vi "Test In-Range ARGB Image.vi"(8 "error in (no error)":errorcluster, 11 "Test Case In":refnum<class "01_Image.lvclass">) -> (0 "error out":errorcluster, 3 "Test Case Out":refnum<class "01_Image.lvclass">)   [LabVIEW 2020, in "test.lvlib" / "01_Image.lvclass"]
uses:
  01_Image.lvclass
  C:/Program Files (x86)/National Instruments/LabVIEW 2026/vi.lib/Astemes/LUnit/Test Case.lvclass
  common/Image Size (Integer).ctl
  image/In-Range Image Colour Range.ctl
  <vilib>/Astemes/LUnit/Test Case.lvclass/Test Case.ctl
  image/New Image (Greyscale Preallocated).vi
  4993e8ee-a06a-463a-9684-69129f64d5ce.vi
  image/New Image (ARGB Preallocated).vi
  image/Copy Array to Image.vi
  image/Copy Array to Image (ARGB).vi
  image/New Image (Greyscale Preallocated).vi/6598b9e0-8a08-46f5-91fd-ca1b87217137.vi
  image/In-Range (ARGB).vi/ffccc43a-a069-4092-9152-56f2c6e40fec.vi
  <vilib>/Astemes/LUnit/Core/LUnit Test Case/Private/Append Pass Result.vi
  <vilib>/Astemes/LUnit/Core/LUnit Test Case/Private/Append Fail Result.vi
  4993e8ee-a06a-463a-9684-69129f64d5ce.vi/9c5d11cd-9439-4240-a1ee-d9baace9c924.vi
  image/New Image (ARGB Preallocated).vi/3321fa97-f432-4e1e-8db9-a0df79aed21b.vi
  image/ARGB Colour to U32 Pixel Value.vi
  <vilib>/Astemes/LUnit/Core/LUnit Test Case/Private/Run In UI.vi
  <vilib>/Utility/error.llb/Clear Errors.vi
  <vilib>/Utility/error.llb/Error Cluster From Error Code.vi
  <vilib>/picture/pixmap.llb/Flatten Pixmap.vi
  image/image.lvlib
  common/common.lvlib
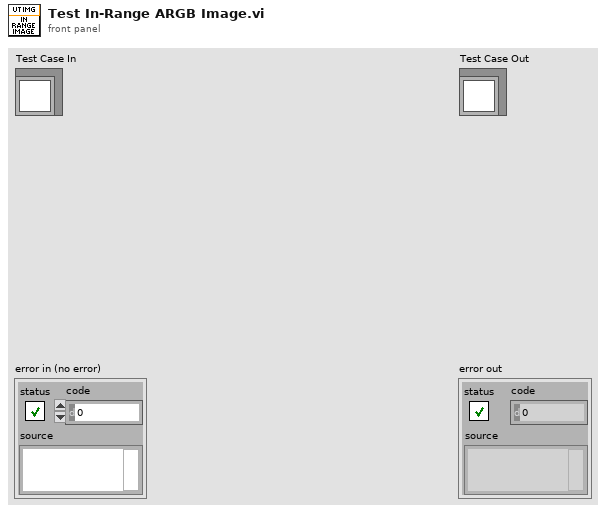
[diagram p1: front panel]
types:
  T1 = typedef "image.lvlib/In-Range Image Colour Range.ctl" = cluster{"Lower":u32, "Upper":u32}
  T2 = typedef "common.lvlib/Image Size (Integer).ctl" = cluster{"Width":u16, "Height":u16}
  T3 = typedef "image.lvlib/ARGB Image.ctl" = refnum<data-value>
  T4 = typedef "image.lvlib/Greyscale Image.ctl" = refnum<data-value>
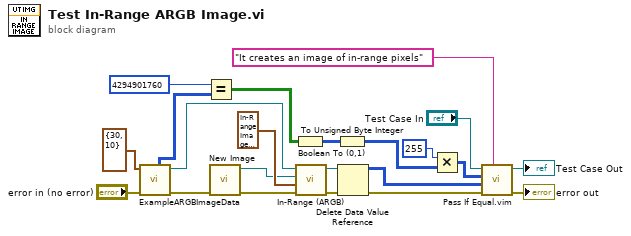
[diagram p0: block diagram]
diagram:
  n1 = call "ExampleARGBImageData.vi"("error in (no error)"="error in (no error)", "Image Size"=T2 {"Width"=30, "Height"=10} ("Preallocated Image Size (Default - 0,0)")) -> ("error out"=w17:errorcluster, "Data Value Reference out"=w11:T3, "ARGB Array Data"=w10:u32[][])  [unwired: 6 in, 1 out]
  n2 = Equal?(x=u32 4294901760 ("color(black)"), y=w10) -> (x = y?=w8:bool[][])
  n3 = call-poly "New Image.vi"("error in (no error)"=w17) -> ("error out"=w16:errorcluster, "Greyscale Image"=w12:T4)  [unwired: 9 in]
  n4 = Boolean To (0,1)(Boolean=w8) -> (0, 1=w7:i16[][])
  n5 = call "In-Range (ARGB).vi"("error in (no error)"=w16, "In-Range Image Colour Range"=T1 {"Lower"=16711680, "Upper"=16760576}, "In-Range-Result in"=w12, "ARGB Image Source in"=w11) -> ("error out"=w13:errorcluster, "In-Range-Result"=w4:T4)  [unwired: 6 in]
  n6 = To Unsigned Byte Integer(number=w7) -> (unsigned 8bit integer=w6:u8[][])
  n7 = Delete Data Value Reference(data value reference=w4, error in=w13) -> (data value=w2:u8[][], error out=w3:errorcluster)
  n8 = Multiply(x=u8 255, y=w6) -> (x*y=w1:u8[][])
  n9 = call "Pass If Equal.vim"("Description"="It creates an image of in-range pixels", "error in (no error)"=w3, "Actual"=w2, "Expected"=w1, "LUnit Test Case In"="Test Case In") -> ("error out"=→"error out":errorcluster, "LUnit Test Case Out"=→"Test Case Out":refnum<class "01_Image.lvclass">)  [unwired: 5 in]
